vi "Self-Test.vi"(8 "error in (no error)":errorcluster, 11 "VISA resource name":refnum<visa-resource-name>) -> (0 "error out":errorcluster, 1 "Self-Test Result Message":string, 2 "Self-Test Result Code":i32, 3 "VISA resource name out":refnum<visa-resource-name>)   [LabVIEW 2020, in "RIGOL DP1000 Series.lvlib"]
doc: "Runs the instrument's self-test routine and returns the test results."
uses:
  <instrlib>/RIGOL DP1000 Series/RIGOL DP1000 Series.lvlib
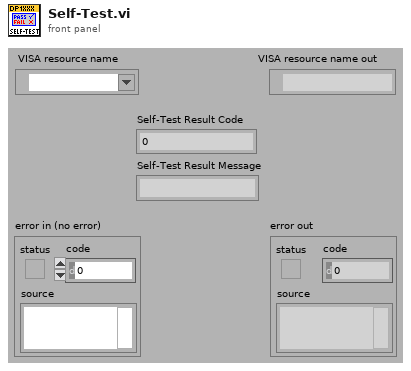
[diagram p1: front panel]
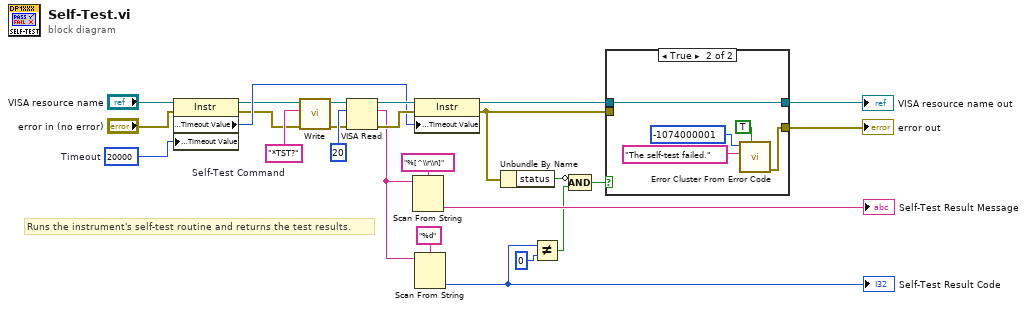
[diagram p0: block diagram]
diagram:
  w16 = u32 20000  # Timeout
  w2 = "*TST?"  # Self-Test Command
  # "Runs the instrument's self-test routine and returns the test results."
  n1 = property class="Instr"(reference="VISA resource name", error in="error in (no error)", "General Settings:Timeout Value"=w16) -> (reference out=w3:refnum<visa-resource-name>, error out=w1:errorcluster, "General Settings:Timeout Value"=w15:u32)
  n2 = call <instrlib>:"Write.vi"("error in (no error)"=w1, "Write Buffer (\"\")"=w2, "VISA resource name"=w3) -> ("error out"=w5:errorcluster, "VISA resource name out"=w4:refnum<visa-resource-name>)  [unwired: 7 in]
  n3 = VISA Read(VISA resource name=w4, byte count=u32 20 ("byte count (20)"), error in (no error)=w5) -> (VISA resource name out=w23:refnum<visa-resource-name>, read buffer=w18:string, error out=w22:errorcluster)  [unwired: 1 out]
  n4 = Scan From String(format string="%[^\\r\\n]" ("Format String"), input string=w18) -> (output 1=→"Self-Test Result Message":string)  [unwired: 2 in, 4 out]
  n5 = property class="Instr"(reference=w23, error in=w22, "General Settings:Timeout Value"=w15) -> (reference out=w14:refnum<visa-resource-name>, error out=w13:errorcluster)
  n6 = Scan From String(format string="%d", input string=w18) -> (output 1=w9:i32)  [unwired: 2 in, 4 out]
  "Self-Test Result Code" <- w9
  n7 = Unbundle By Name(w13) -> ("status"=w11:bool)
  n8 = Not Equal?(x=w9, y=0) -> (x != y?=w12:bool)
  n9 = Compound Arithmetic op=AND(invert w11, w12) -> (w10:bool)
  n10 = case shown="True" w10 {
    tunnel: w14 -> [w27 w32]
    tunnel: w13 -> [w26 _]
    tunnel: [w26 w28] -> w6
    tunnel: [w27 w32] -> w7
    frame False {
    }
    frame True {
      n11 = call <vilib>:"Error Cluster From Error Code.vi"("show call chain? (False)"=TRUE, "error message (\"\")"="The self-test failed." ("Source (VI Name)"), "error code (0)"=-1074000001 ("Code")) -> ("error out"=w28:errorcluster)  [unwired: 1 in, 5 out]
    }
  }
  "VISA resource name out" <- w7
  "error out" <- w6
